vi "String_to_Pathname.vi"(1 "Input String":string) -> (0 "path":path)   [LabVIEW 2011]
uses:
  Globals/Preference_global.vi
  Globals/Constants_global.vi
panel:
  out "size(s)":i32
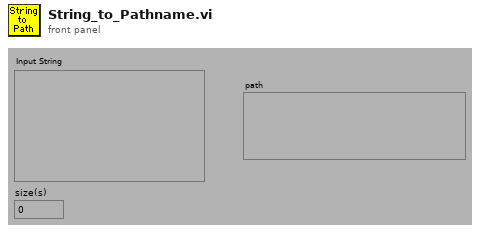
[diagram p1: front panel]
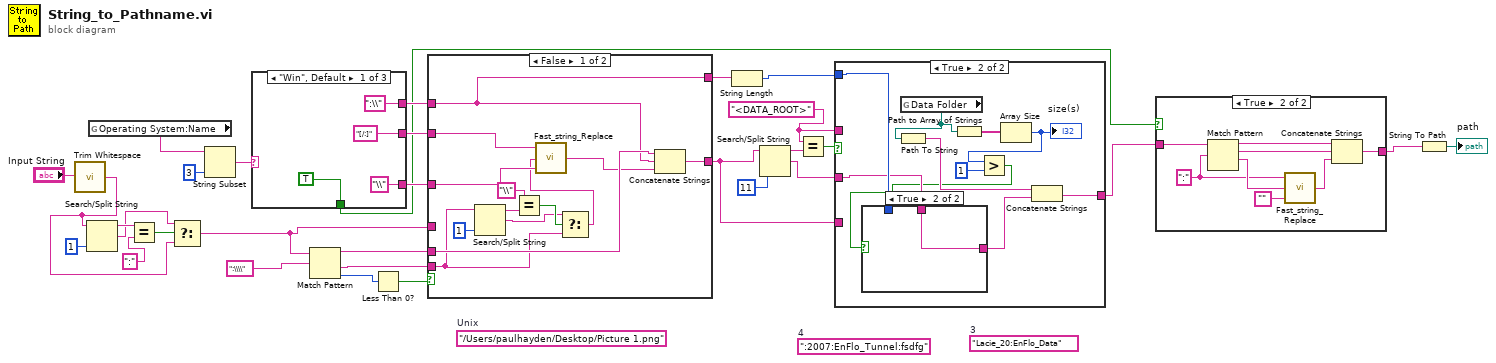
[diagram p0: block diagram]
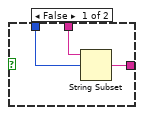
[diagram p4: hidden frame]
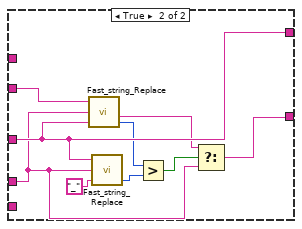
[diagram p5: hidden frame]
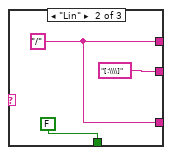
[diagram p6: hidden frame]
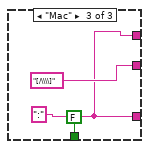
[diagram p7: hidden frame]
diagram:
  (unwired) "Lacie_20:EnFlo_Data"  # 3
  (unwired) ":2007:EnFlo_Tunnel:fsdfg"  # 4
  (unwired) "/Users/paulhayden/Desktop/Picture 1.png"  # Unix
  w11 = "<DATA_ROOT>" ("regular expression")
  n1 = call <vilib>:"Trim Whitespace.vi"("string"="Input String") -> ("trimmed string"=w4:string)  [unwired: 1 in]
  n2 = Search/Split String(string=w4, offset (0)=1 ("length (rest)")) -> (substring before match=w20:string, match + rest of string=w19:string)  [unwired: 2 out]
  n3 = global read "Preference_global.vi" "Operating System:Name"() -> (w30:string)
  n4 = Equal?(x=w20, y=":") -> (x = y?=w22:bool)
  n5 = Select(t=w19, s=w22, f=w4) -> (s? t:f=w18:string)
  n6 = String Subset(string=w30, length (rest)=3 ("length (rest)")) -> (substring=w31:string)  [unwired: 1 out]
  n7 = case shown="\"Win\", Default" w31 {
    tunnel: ["[/:]" "[:\\\\]" "[/\\\\]"] -> w25
    tunnel: ["\\" w37 w40] -> w24
    tunnel: [":\\" w37 w40] -> w9
    tunnel: [TRUE FALSE FALSE] -> w1
    frame "Win", Default {
    }
    frame "Lin" {
      w37 = "/"
    }
    frame "Mac" {
      w40 = ":"
    }
  }
  n8 = Match Pattern(string=w18, regular expression=":\\\\") -> (before substring=w16:string, after substring=w17:string, offset past match=w27:i32)  [unwired: 2 out]
  n9 = Less Than 0?(x=w27) -> (x < 0?=w26:bool)
  n10 = case shown="False" w26 {
    tunnel: w18 -> [_ w56]
    tunnel: w25 -> [w54 w63]
    tunnel: w24 -> [w53 w62]
    tunnel: w17 -> [w43 _]
    tunnel: w16 -> [w52 _]
    tunnel: w9 -> [w49 _]
    tunnel: [w50 w55] -> w13
    tunnel: [w49 w62] -> w6
    frame False {
      n11 = Search/Split String(string=w43, offset (0)=1 ("length (rest)")) -> (substring before match=w47:string, match + rest of string=w44:string)  [unwired: 2 out]
      n12 = Equal?(x="\\", y=w47) -> (x = y?=w45:bool)
      n13 = Select(t=w44, s=w45, f=w43) -> (s? t:f=w42:string)
      n14 = call "Fast_string_Replace.vi"("Replace match with:"=w53, "Input String"=w42, "regular expression"=w54) -> ("Output String"=w51:string)  [unwired: 2 out]
      n15 = Concatenate Strings(w52, w49, w51) -> (w50:string)
    }
    frame True {
      n16 = call "Fast_string_Replace.vi"("Replace match with:"=w62, "Input String"=w56, "regular expression"=w63) -> ("Number Found"=w60:i32, "Output String"=w57:string)  [unwired: 1 out]
      n17 = call "Fast_string_Replace.vi"("Replace match with:"="_", "Input String"=w56, "regular expression"=w62) -> ("Number Found"=w59:i32)  [unwired: 2 out]
      n18 = Greater?(x=w60, y=w59) -> (0:w58:bool)
      n19 = Select(t=w57, s=w58, f=w56) -> (s? t:f=w55:string)
    }
  }
  n20 = String Length(string=w6) -> (length=w7:i32)
  n21 = Search/Split String(string=w13, offset (0)=11) -> (substring before match=w15:string, match + rest of string=w10:string)  [unwired: 1 in, 1 out]
  n22 = Equal?(x=w11, y=w15) -> (x = y?=w14:bool)
  n23 = case shown="True" w14 {
    tunnel: w13 -> [w64 _]
    tunnel: [w64 w68] -> w3
    tunnel: w11 -> [_ _]
    tunnel: w10 -> [_ w72]
    tunnel: w7 -> [_ w73]
    frame False {
    }
    frame True {
      n24 = global read "Constants_global.vi" "Data Folder"() -> (w70:path)
      n25 = Path To String(path=w70) -> (string=w74:string)
      n26 = Path to Array of Strings(0:w70) -> (2:w69:string[])  [unwired: 1 out]
      n27 = Array Size(array=w69) -> (size(s)=w67:i32)
      "size(s)" <- w67
      n28 = Greater?(x=w67, y=1) -> (0:w65:bool)
      n29 = case shown="True" w65 {
        tunnel: w73 -> [w77 _]
        tunnel: w72 -> [w76 w78]
        tunnel: [w75 w78] -> w71
        frame False {
          n30 = String Subset(string=w76, offset (0)=w77) -> (substring=w75:string)  [unwired: 1 out]
        }
        frame True {
        }
      }
      n31 = Concatenate Strings(w74, w71) -> (w68:string)
    }
  }
  n32 = case shown="True" w1 {
    tunnel: w3 -> [w79 w87]
    tunnel: [w79 w80] -> w2
    frame False {
    }
    frame True {
      w85 = ":" ("regular expression")
      n33 = Match Pattern(string=w87, regular expression=w85) -> (before substring=w82:string, match substring=w81:string, after substring=w86:string)  [unwired: 2 out]
      n34 = call "Fast_string_Replace.vi"("Replace match with:"="", "Input String"=w86, "regular expression"=w85) -> ("Output String"=w83:string)  [unwired: 2 out]
      n35 = Concatenate Strings(w82, w81, w83) -> (w80:string)
    }
  }
  n36 = String To Path(string=w2) -> (path=→"path":path)
